vi "To Default Object.vi"(11 "Object in":refnum<class>) -> (3 "Default out":refnum<class>)   [LabVIEW 2020]
doc: "Restore 'Object in' to the default value by using preserve run tim class."
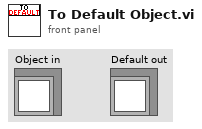
[diagram p1: front panel]
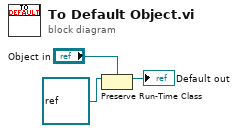
[diagram p0: block diagram]
diagram:
  n1 = Preserve Run-Time Class(object in=refnum<class> refnum, 2:"Object in") -> (object out=→"Default out":refnum<class>)  [unwired: 1 in, 1 out]
